vi "verificator de eroare.vi"() -> ()   [LabVIEW 2019]
panel:
  out "Mesaj Corupt":bool
  in  "String 2":string
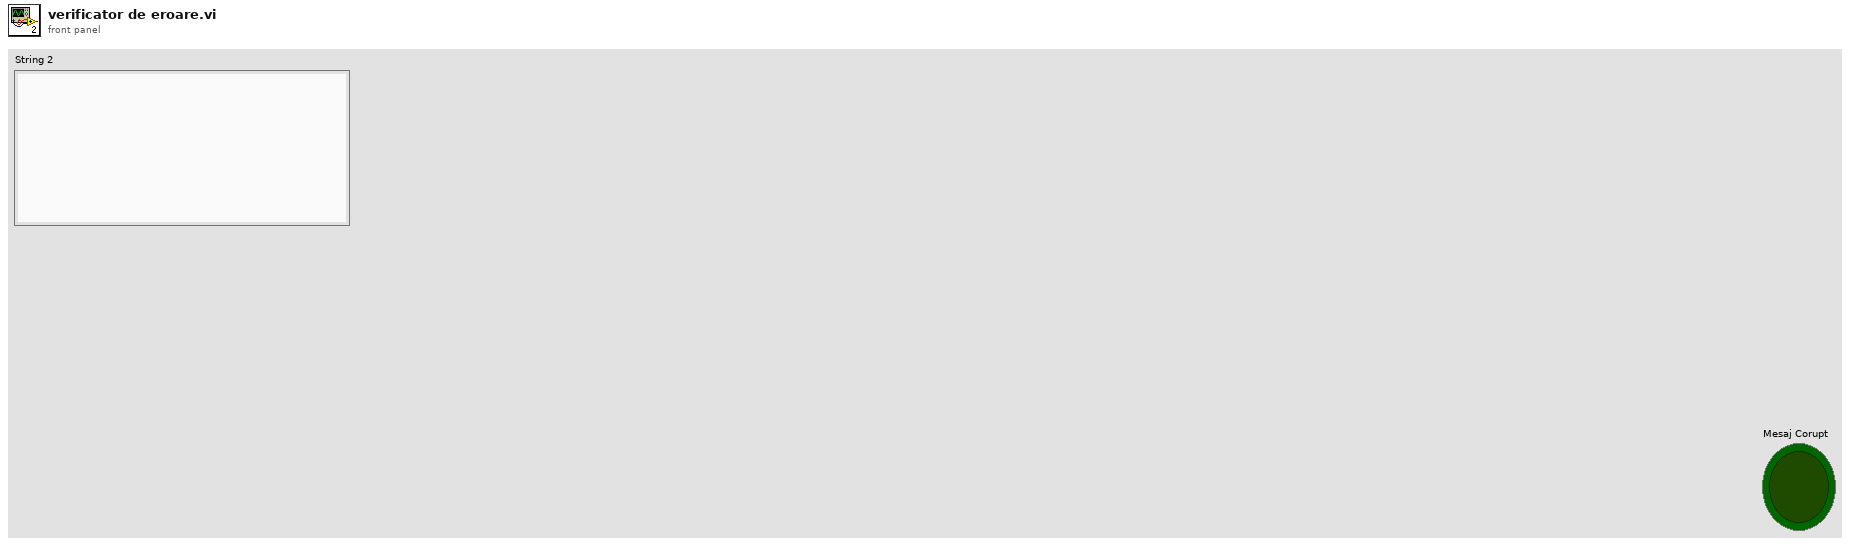
[diagram p1: front panel]
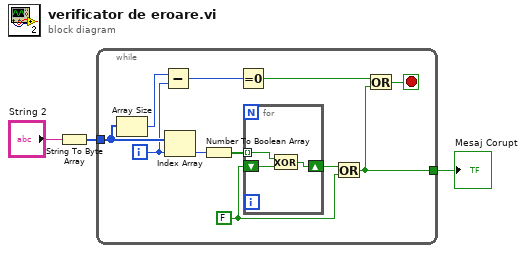
[diagram p0: block diagram]
diagram:
  n1 = String To Byte Array(string="String 2") -> (unsigned byte array=w2:u8[])
  n2 = while {
    tunnel: w2 -> [w14]
    tunnel: [w4] -> w1
    i -> [w9]
    stop <- w5 stop-if-true
    w7 = FALSE
    n3 = Array Size(array=w14) -> (size(s)=w13:i32)
    n4 = Subtract(x=w13, y=w9) -> (x-y=w12:i32)
    n5 = Index Array(array=w14, index=w9) -> (element=w11:u8)
    n6 = Number To Boolean Array(number=w11) -> (Boolean array=w10:bool[])
    n7 = Equal To 0?(x=w12) -> (x = 0?=w6:bool)
    n8 = for {
      tunnel: w10 -> [w15] mode=indexing
      shift-right: [w16] -> w8
      shift-left: w7 -> [w17]
      n9 = Exclusive Or(1:w17, 2:w15) -> (0:w16:bool)
    }
    n10 = Or(x=w8, y=w7) -> (x .or. y?=w4:bool)
    n11 = Or(x=w6, y=w4) -> (x .or. y?=w5:bool)
  }
  "Mesaj Corupt" <- w1
